vi "Extract the same PlayerID Channels.vi"(8 "error in (no error)":errorcluster, 11 "Channel Refs in":T1[](array[typedef]) format="%.0x") -> (0 "error out":errorcluster, 1 "PlayerID":u8, 2 "Extracted the same PlayerID Channel Refs":T1[](array[typedef]) format="%.0x", 3 "Channel Refs Remaining":T1[](array[typedef]) format="%.0x")   [LabVIEW 2023, in "Vires VTD System Explorer.lvlib"]
uses:
  Vires VTD System Explorer.lvlib
  <vilib>/NI VeriStand/Custom Device API/Custom Device Item Ref.ctl
  <vilib>/NI VeriStand/Custom Device API/Get Item Property (Variant).vi
  <vilib>/NI VeriStand/Custom Device API/Custom Device API.lvlib
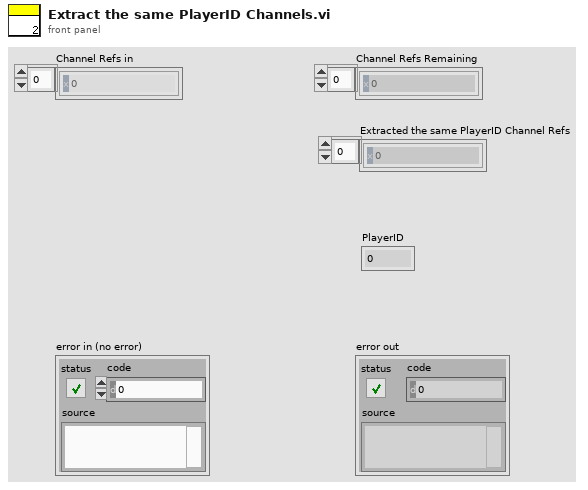
[diagram p1: front panel]
types:
  T1 = typedef "Custom Device API.lvlib/Custom Device Item Ref.ctl" = u64
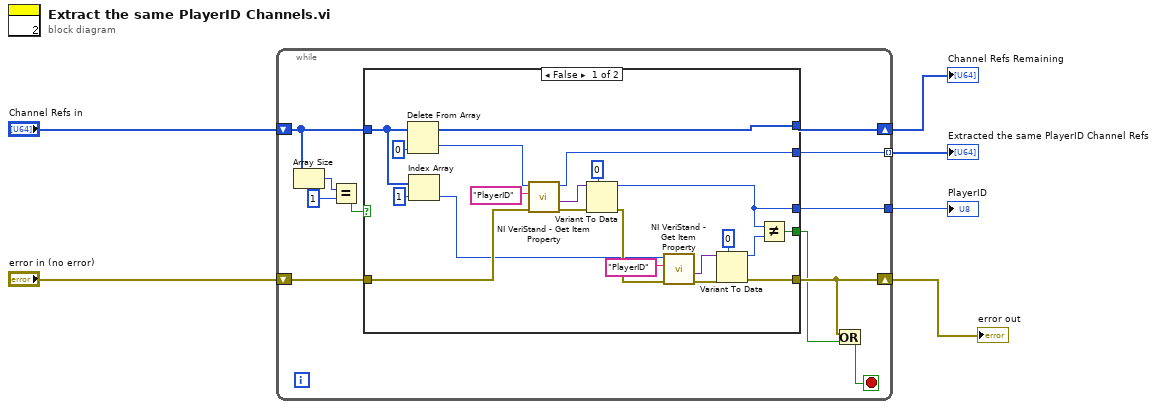
[diagram p0: block diagram]
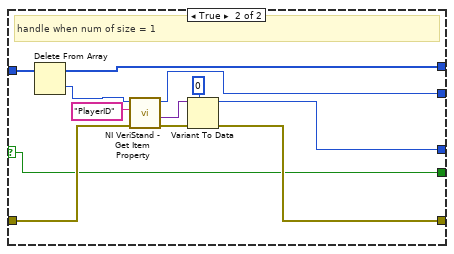
[diagram p2: hidden frame]
diagram:
  n1 = while {
    shift-right: [w9] -> w4
    shift-left: "error in (no error)" -> [w17]
    tunnel: [w16] -> w3 mode=indexing
    tunnel: [w15] -> w5
    shift-right: [w10] -> w6
    shift-left: "Channel Refs in" -> [w12]
    stop <- w7 stop-if-true
    n2 = Array Size(array=w12) -> (size(s)=w13:i32)
    n3 = Equal?(x=w13, y=1) -> (x = y?=w11:bool)
    n4 = case shown="False" w11 {
      selector: w11 -> [_ w44]
      tunnel: [w31 w45] -> w9
      tunnel: w17 -> [w30 w46]
      tunnel: [w26 w44] -> w8
      tunnel: [w25 w43] -> w16
      tunnel: [w24 w42] -> w15
      tunnel: w12 -> [w23 w41]
      tunnel: [w18 w40] -> w10
      frame False {
        n5 = Delete From Array(array=w23, index=0) -> (deleted portion=w19:T1, array with subset deleted=w18:T1[])  [unwired: 1 in]
        n6 = Index Array(array=w23, index=1) -> (element=w22:T1)
        n7 = call-poly <vilib>:"NI VeriStand - Get Item Property.vi"("error in (no error)"=w30, "Property Name"="PlayerID", "Item Ref in"=w19) -> ("error out"=w36:errorcluster, "Value"=w35:variant, "Item Ref out"=w25:T1)  [unwired: 5 in, 1 out]
        n8 = Variant To Data(error in=w36, type=u8 0, Variant=w35) -> (data=w24:u8, error out=w34:errorcluster)
        n9 = call-poly <vilib>:"NI VeriStand - Get Item Property.vi"("error in (no error)"=w34, "Property Name"="PlayerID", "Item Ref in"=w22) -> ("error out"=w33:errorcluster, "Value"=w32:variant)  [unwired: 5 in, 2 out]
        n10 = Variant To Data(error in=w33, type=u8 0, Variant=w32) -> (data=w28:u8, error out=w31:errorcluster)
        n11 = Not Equal?(x=w24, y=w28) -> (x != y?=w26:bool)
      }
      frame True {
        # "handle when num of size = 1"
        n12 = Delete From Array(array=w41) -> (deleted portion=w39:T1, array with subset deleted=w40:T1[])  [unwired: 2 in]
        n13 = call-poly <vilib>:"NI VeriStand - Get Item Property.vi"("error in (no error)"=w46, "Property Name"="PlayerID", "Item Ref in"=w39) -> ("error out"=w48:errorcluster, "Value"=w49:variant, "Item Ref out"=w43:T1)  [unwired: 5 in, 1 out]
        n14 = Variant To Data(error in=w48, type=u8 0, Variant=w49) -> (data=w42:u8, error out=w45:errorcluster)
      }
    }
    n15 = Or(x=w9, y=w8) -> (x .or. y?=w7:bool)
  }
  "Channel Refs Remaining" <- w6
  "PlayerID" <- w5
  "error out" <- w4
  "Extracted the same PlayerID Channel Refs" <- w3
